vi "Read Laser.vi"(8 "error in (no error)":errorcluster, 11 "CRDS Cell in":refnum<class "CRDS Cell.lvclass">) -> (0 "error out":errorcluster, 2 "Laser":T1=enum."Blue", 3 "CRDS Cell out":refnum<class "CRDS Cell.lvclass">)   [LabVIEW 2011]
doc: "Retrieve the wavelength descriptor. This can be blue, green or red, the color of the laser."
uses:
  CRDS Cell.lvclass
  PAS_CRDS new/CRDS/Controls/las_lambda.ctl
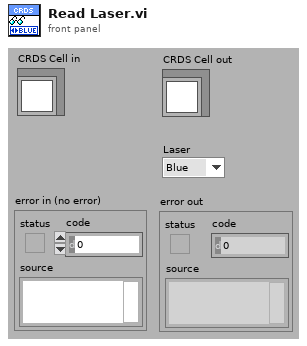
[diagram p1: front panel]
types:
  T1 = typedef "las_lambda.ctl" = enum16{"Red", "Blue", "Green"}
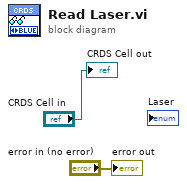
[diagram p0: block diagram]
diagram:
  "error out" <- "error in (no error)"
  "CRDS Cell out" <- "CRDS Cell in"
